vi "end.vi"(8 "error in (no error)":errorcluster, 11 "Save Image in":refnum<class "Save Image.lvclass">) -> (0 "error out":errorcluster, 3 "Save Image out":refnum<class "Save Image.lvclass">)   [LabVIEW 2018, in "Save Image.lvclass"]
doc: "End the Python Toolkit correctly"
uses:
  Save Image.lvclass
  Save Image.lvclass/Save Image.ctl
  Python Toolkit/Python Toolkit.lvclass
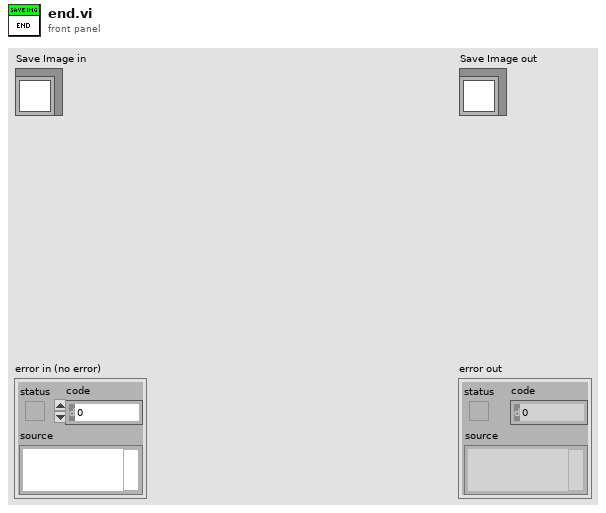
[diagram p1: front panel]
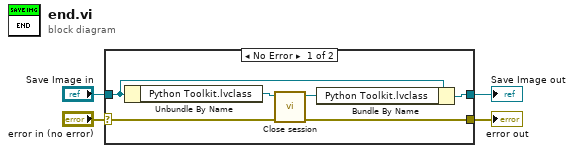
[diagram p0: block diagram]
diagram:
  n1 = case shown="No Error" "error in (no error)" {
    selector: "error in (no error)" -> [w8 w12]
    tunnel: [w5 w12] -> w3
    tunnel: [w9 w11] -> w1
    tunnel: "Save Image in" -> [w10 w11]
    frame No Error {
      n2 = Unbundle By Name(w10) -> ("Python Toolkit.lvclass"=w7:refnum<class "Python Toolkit.lvclass">)
      n3 = call "Close session.vi"("error in (no error)"=w8, "Python Toolkit in"=w7) -> ("error out"=w5:errorcluster, "Python Toolkit out"=w6:refnum<class "Python Toolkit.lvclass">)  [unwired: 8 in]
      n4 = Bundle By Name(cluster=w10, "Python Toolkit.lvclass"=w6) -> (w9:refnum<class "Save Image.lvclass">)
    }
    frame Error {
    }
  }
  "error out" <- w3
  "Save Image out" <- w1
